vi "PFD_VerticalSpeed.vi"(8 "Refresh Rate (Hz)":u32=30) -> ()   [LabVIEW 2023]
uses:
  <vilib>/Utility/miscctls.llb/LVBoundsTypeDef.ctl
  <vilib>/picture/picture.llb/imagedata.ctl
  pfd_global.vi
panel:
  out "x .or. y?":bool
  out "PFD_VerticalControl":sgl
  out "PFD_Vertical":picture
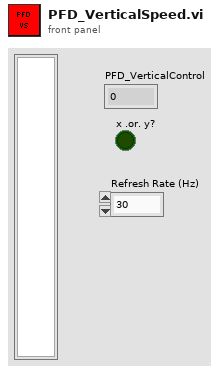
[diagram p1: front panel]
types:
  T1 = typedef "LVBoundsTypeDef.ctl" = cluster{"Width":u32, "Height":u32}
  T2 = cluster{"Width":u16, "Style":enum32{"Solid", "Dash", "Dot", "DashDot", "DashDotDot"}}
  T3 = cluster{"left":i16, "top":i16, "right":i16, "bottom":i16}
  T4 = typedef "imagedata.ctl" = cluster{"image type":i32, "image depth":i32, "image":u8[], "mask":u8[], "colors":u32[], "Rectangle":cluster{"left":i16, "top":i16, "right":i16, "bottom":i16}}
  T5 = cluster{"horizontal":enum16{"left", "center", "right"}, "vertical":enum16{"top", "center", "bottom"}}
  T6 = cluster{"Font Name:":string, "Size":i16, "Strikeout?":bool, "Italic?":bool, "Underline?":bool, "Outline?":bool, "Shadow?":bool, "Bold?":bool}
  T7 = enum16{"User-specified Font", "Application Font", "System Font", "Dialog Font"}
  T8 = cluster{cluster{i16, i16}, "output cluster":cluster{i16, i16}}
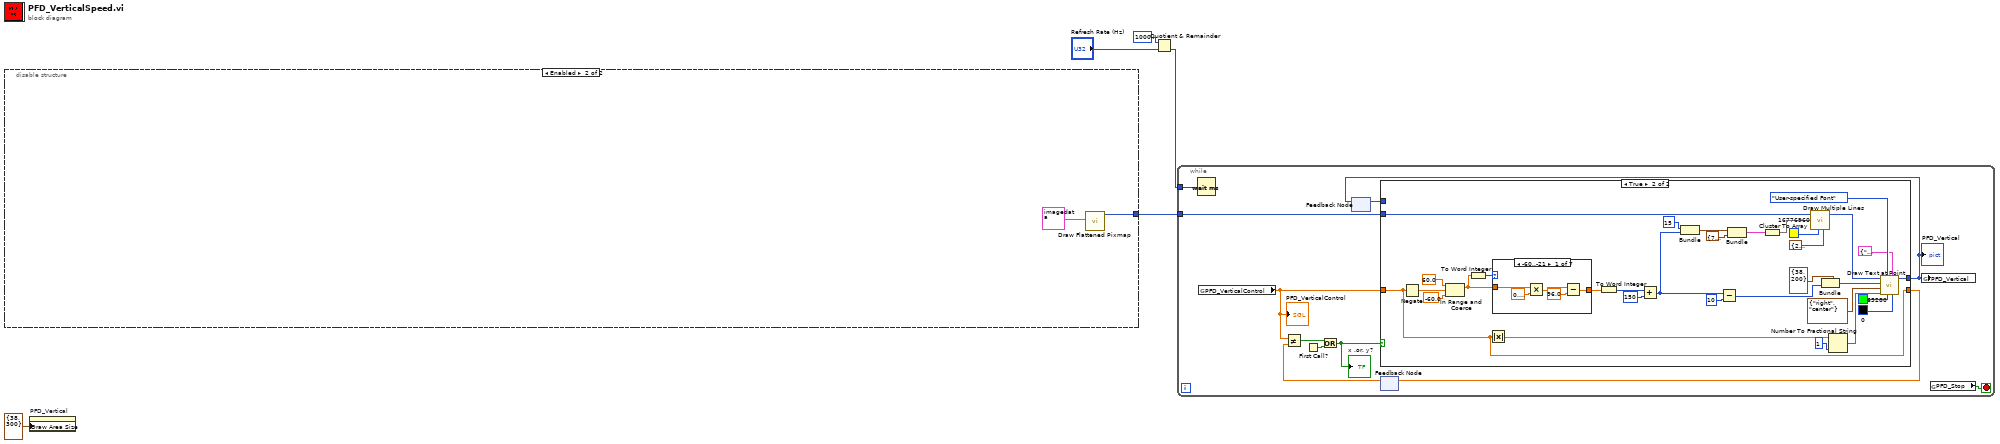
[diagram p0: block diagram]
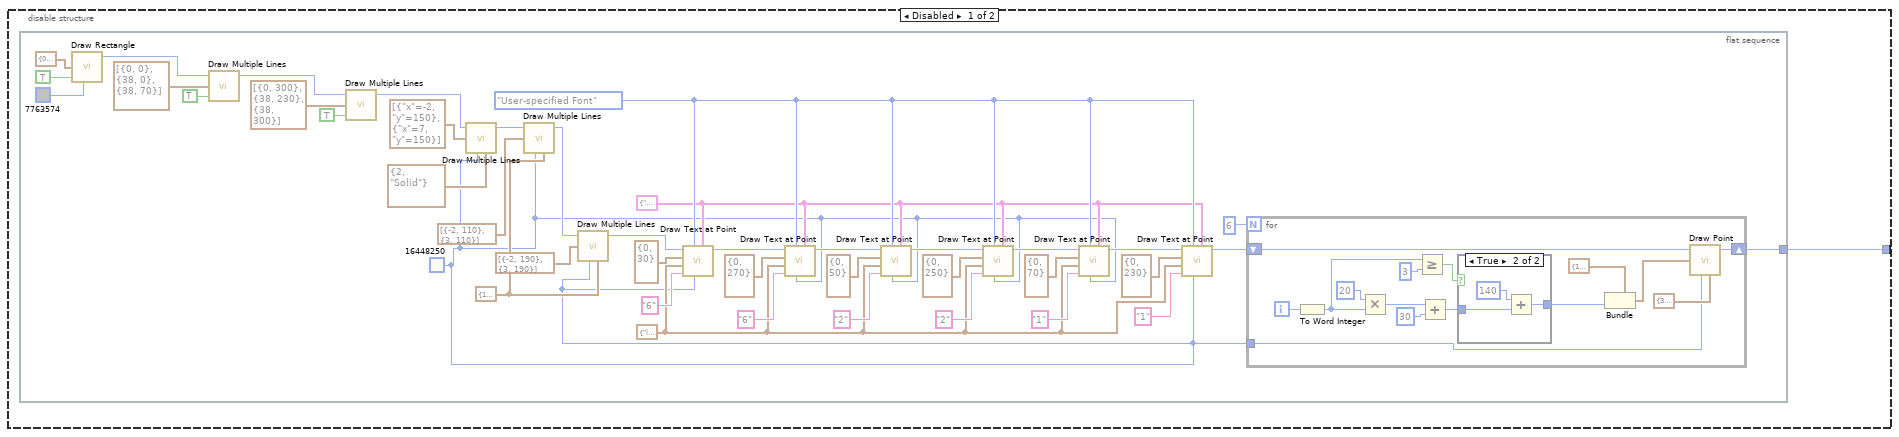
[diagram p2: hidden frame]
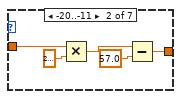
[diagram p5: hidden frame]
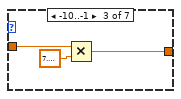
[diagram p6: hidden frame]
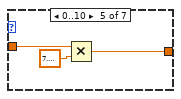
[diagram p8: hidden frame]
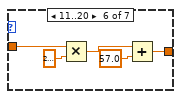
[diagram p9: hidden frame]
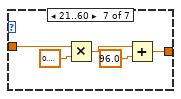
[diagram p10: hidden frame]
diagram:
  n1 = disable-structure shown="Enabled" {
    disable-tunnel: [w6 w69] -> w5
    frame Disabled {
      n2 = flat-sequence {
        tunnel: [w8] -> w6
        frame #0 {
          w10 = u32 16448250 ("color(black)")
          w14 = T5 {"horizontal"=enum."left", "vertical"=enum."center"} ("alignment(left, top)")
          w15 = T6 {"Font Name:"="vspeed", "Size"=15, "Strikeout?"=FALSE, "Italic?"=FALSE, "Underline?"=FALSE, "Outline?"=FALSE, "Shadow?"=FALSE, "Bold?"=TRUE} ("[user-specified font]")
          w16 = T7."User-specified Font" ("desired font(Application)")
          w34 = T2 {"Width"=1, "Style"=enum."Solid"} ("pen")
          n3 = call <vilib>:"Draw Rectangle.vi"("rect"=T3 {"left"=0, "top"=0, "right"=38, "bottom"=300}, "fill?(F)"=TRUE, "color(black)"=u32 7763574 ("Speed_color_background")) -> ("new picture"=w47:picture)  [unwired: 6 in]
          n4 = call <vilib>:"Draw Multiple Lines.vi"("picture"=w47, "line endpoints"=cluster{"x":i16, "y":i16}[] [{"x"=0, "y"=0}, {"x"=38, "y"=0}, {"x"=38, "y"=70}], "fill?(F)"=TRUE) -> ("new picture"=w43:picture)  [unwired: 6 in]
          n5 = call <vilib>:"Draw Multiple Lines.vi"("picture"=w43, "line endpoints"=cluster{"x":i16, "y":i16}[] [{"x"=0, "y"=300}, {"x"=38, "y"=230}, {"x"=38, "y"=300}] ("line endpoints 2"), "fill?(F)"=TRUE) -> ("new picture"=w40:picture)  [unwired: 6 in]
          n6 = call <vilib>:"Draw Multiple Lines.vi"("picture"=w40, "line endpoints"=cluster{"x":i16, "y":i16}[] [{"x"=-2, "y"=150}, {"x"=7, "y"=150}], "color(black)"=w10, "pen"=T2 {"Width"=2, "Style"=enum."Solid"}) -> ("new picture"=w39:picture)  [unwired: 5 in]
          n7 = call <vilib>:"Draw Multiple Lines.vi"("picture"=w39, "line endpoints"=cluster{"x":i16, "y":i16}[] [{"x"=-2, "y"=110}, {"x"=3, "y"=110}] ("line endpoints 2"), "color(black)"=w10, "pen"=w34) -> ("new picture"=w35:picture)  [unwired: 5 in]
          n8 = call <vilib>:"Draw Multiple Lines.vi"("picture"=w35, "line endpoints"=cluster{"x":i16, "y":i16}[] [{"x"=-2, "y"=190}, {"x"=3, "y"=190}] ("line endpoints 3"), "color(black)"=w10, "pen"=w34) -> ("new picture"=w32:picture)  [unwired: 5 in]
          n9 = call <vilib>:"Draw Text at Point.vi"("[user-specified font]"=w15, "text color(black)"=w10, "desired font(Application)"=w16, "text"="6", "alignment(left, top)"=w14, "origin"=cluster{"x":i16, "y":i16} {"x"=0, "y"=30} ("origin 3"), "picture"=w32) -> ("new picture"=w29:picture)  [unwired: 3 in, 1 out]
          n10 = call <vilib>:"Draw Text at Point.vi"("[user-specified font]"=w15, "text color(black)"=w10, "desired font(Application)"=w16, "text"="6", "alignment(left, top)"=w14, "origin"=cluster{"x":i16, "y":i16} {"x"=0, "y"=270} ("origin 2"), "picture"=w29) -> ("new picture"=w26:picture)  [unwired: 3 in, 1 out]
          n11 = call <vilib>:"Draw Text at Point.vi"("[user-specified font]"=w15, "text color(black)"=w10, "desired font(Application)"=w16, "text"="2", "alignment(left, top)"=w14, "origin"=cluster{"x":i16, "y":i16} {"x"=0, "y"=50} ("origin 3"), "picture"=w26) -> ("new picture"=w23:picture)  [unwired: 3 in, 1 out]
          n12 = call <vilib>:"Draw Text at Point.vi"("[user-specified font]"=w15, "text color(black)"=w10, "desired font(Application)"=w16, "text"="2", "alignment(left, top)"=w14, "origin"=cluster{"x":i16, "y":i16} {"x"=0, "y"=250}, "picture"=w23) -> ("new picture"=w21:picture)  [unwired: 3 in, 1 out]
          n13 = call <vilib>:"Draw Text at Point.vi"("[user-specified font]"=w15, "text color(black)"=w10, "desired font(Application)"=w16, "text"="1", "alignment(left, top)"=w14, "origin"=cluster{"x":i16, "y":i16} {"x"=0, "y"=70} ("origin 2"), "picture"=w21) -> ("new picture"=w17:picture)  [unwired: 3 in, 1 out]
          n14 = call <vilib>:"Draw Text at Point.vi"("[user-specified font]"=w15, "text color(black)"=w10, "desired font(Application)"=w16, "text"="1", "alignment(left, top)"=w14, "origin"=cluster{"x":i16, "y":i16} {"x"=0, "y"=230} ("origin 4"), "picture"=w17) -> ("new picture"=w11:picture)  [unwired: 3 in, 1 out]
          n15 = for {
            N: 6 -> [_]
            tunnel: w10 -> [w60]
            shift-right: [w62] -> w8
            shift-left: w11 -> [w63]
            i -> [w57]
            n16 = To Word Integer(number=w57) -> (16bit integer=w52:i16)
            n17 = Multiply(x=i16 20, y=w52) -> (x*y=w55:i16)
            n18 = Greater Or Equal?(x=w52, y=i16 3) -> (x >= y?=w53:bool)
            n19 = Add(x=w55, y=i16 30) -> (x+y=w50:i16)
            n20 = case shown="True" w53 {
              tunnel: w50 -> [w64 w67]
              tunnel: [w64 w65] -> w49
              frame False {
              }
              frame True {
                n21 = Add(x=i16 140, y=w67) -> (x+y=w65:i16)
              }
            }
            n22 = Bundle(cluster=cluster{"x":i16, "y":i16} {"x"=10, "y"=30} ("point(x,y)"), "y"=w49) -> (w58:cluster{"x":i16, "y":i16})  [unwired: 1 in]
            n23 = call <vilib>:"Draw Point.vi"("picture"=w63, "point(x,y)"=w58, "color(black)"=w60, "pen"=T2 {"Width"=3, "Style"=enum."Solid"}) -> ("new picture"=w62:picture)  [unwired: 5 in]
          }
        }
      }
    }
    frame Enabled {
      n24 = call <vilib>:"Draw Flattened Pixmap.vi"("image data"=T4 {"image type"=0, "image depth"=24, "image"=array[36000 elements], "mask"=[], "colors"=[], "Rectangle"={"left"=-2, "top"=0, "right"=38, "bottom"=300}}) -> ("new picture"=w69:picture)  [unwired: 8 in]
    }
  }
  n25 = property on="PFD_Vertical" class="Pict"("Draw Area Size"=T1 {"Width"=38, "Height"=300}) -> ()  [unwired: 2 in, 2 out]
  n26 = Quotient & Remainder(x=u32 1000, y="Refresh Rate (Hz)") -> (floor(x/y)=w3:u32)  [unwired: 1 out]
  n27 = while {
    tunnel: w5 -> [w80]
    tunnel: w3 -> [w73]
    stop <- w72 stop-if-true
    n28 = Wait (ms)(milliseconds to wait=w73) -> ()  [unwired: 1 out]
    n29 = global read "pfd_global.vi" "PFD_VerticalControl"() -> (w71:sgl)
    "PFD_VerticalControl" <- w71
    n30 = First Call?() -> (First Call?: T/F=w74:bool)
    n31 = feedback #1() -> (w79:picture)  [unwired: 1 in]
    n32 = feedback #2() -> (w77:sgl)  [unwired: 1 in]
    n33 = Not Equal?(x=w71, y=w77) -> (x != y?=w76:bool)
    n34 = Or(x=w76, y=w74) -> (x .or. y?=w75:bool)
    "x .or. y?" <- w75
    n35 = case shown="True" w75 {
      tunnel: w80 -> [_ w114]
      tunnel: [w82 w83] -> w70
      tunnel: w71 -> [w81 w85]
      tunnel: w79 -> [w82 _]
      tunnel: [w81 w85] -> w78
      frame False {
      }
      frame True {
        n36 = Negate(x=w85) -> (-x=w84:sgl)
        n37 = In Range and Coerce(upper limit=sgl 60.0, x=w84, lower limit=sgl -60.0) -> (coerced(x)=w97:sgl)  [unwired: 1 out]
        n38 = To Word Integer(number=w97) -> (16bit integer=w105:i16)
        n39 = Absolute Value(x=w85) -> (abs(x)=w86:sgl)
        n40 = case shown="-60..-21" w105 {
          tunnel: w97 -> [w118 w123 w126 w128 w130 w135 w140]
          tunnel: [w115 w120 w125 w128 w129 w132 w137] -> w104
          frame -60..-21 {
            n41 = Multiply(x=w118, y=sgl 0.3 ("y 2")) -> (x*y=w117:sgl)
            n42 = Subtract(x=w117, y=sgl 96.0) -> (x-y=w115:sgl)
          }
          frame -20..-11 {
            n43 = Multiply(x=w123, y=sgl 2.0000002) -> (x*y=w122:sgl)
            n44 = Subtract(x=w122, y=sgl 57.0 ("y 3")) -> (x-y=w120:sgl)
          }
          frame -10..-1 {
            n45 = Multiply(x=w126, y=sgl 7.6) -> (x*y=w125:sgl)
          }
          frame 300, Default {
          }
          frame 0..10 {
            n46 = Multiply(x=w130, y=sgl 7.6) -> (x*y=w129:sgl)
          }
          frame 11..20 {
            n47 = Multiply(x=w135, y=sgl 2.0000002) -> (x*y=w134:sgl)
            n48 = Add(x=w134, y=sgl 57.0 ("y 3")) -> (x+y=w132:sgl)
          }
          frame 21..60 {
            n49 = Multiply(x=w140, y=sgl 0.3 ("y 2")) -> (x*y=w139:sgl)
            n50 = Add(x=w139, y=sgl 96.0) -> (x+y=w137:sgl)
          }
        }
        n51 = To Word Integer(number=w104) -> (16bit integer=w103:i16)
        n52 = Add(x=w103, y=i16 150) -> (x+y=w89:i16)
        n53 = Bundle(i16 15, w89) -> (w110:cluster{i16, i16})  [unwired: 1 in]
        n54 = Subtract(x=w89, y=i16 10) -> (x-y=w87:i16)
        n55 = Bundle(w110, "output cluster"=cluster{i16, i16} {76, 150}) -> (w108:T8)  [unwired: 1 in]
        n56 = Cluster To Array(cluster=w108) -> (array=w106:cluster{i16, i16}[])
        n57 = call <vilib>:"Draw Multiple Lines.vi"("picture"=w114, "line endpoints"=w106, "color(black)"=u32 16776960, "pen"=T2 {"Width"=2, "Style"=enum."Solid"}) -> ("new picture"=w100:picture)  [unwired: 5 in]
        n58 = Bundle(cluster=cluster{"x":i16, "y":i16} {"x"=38, "y"=200} ("origin"), "y"=w87) -> (w90:cluster{"x":i16, "y":i16})  [unwired: 1 in]
        n59 = Number To Fractional String(number=w86, precision (6)=i16 1) -> (F-format string=w95:string)  [unwired: 2 in]
        n60 = call <vilib>:"Draw Text at Point.vi"("BG color(transparent)"=u32 0, "[user-specified font]"=T6 {"Font Name:"="vs", "Size"=14, "Strikeout?"=FALSE, "Italic?"=FALSE, "Underline?"=FALSE, "Outline?"=FALSE, "Shadow?"=FALSE, "Bold?"=TRUE}, "text color(black)"=u32 65280, "desired font(Application)"=T7."User-specified Font", "text"=w95, "alignment(left, top)"=T5 {"horizontal"=enum."right", "vertical"=enum."center"}, "origin"=w90, "picture"=w100) -> ("new picture"=w83:picture)  [unwired: 2 in, 1 out]
      }
    }
    "PFD_Vertical" <- w70
    n61 = feedback-in #1(w70) -> ()
    n62 = feedback-in #2(w78) -> ()
    n63 = global write "pfd_global.vi" "PFD_Vertical"(w70) -> ()
    n64 = global read "pfd_global.vi" "PFD_Stop"() -> (w72:bool)
  }
